vi "initialize timing source.vi"(8 "error in":errorcluster, 11 "timing source in":refnum<class "usec timing source.lvclass">) -> (0 "error out":errorcluster, 3 "timing source out":refnum<class "usec timing source.lvclass">)   [LabVIEW 2013, in "usec timing source.lvclass"]
doc: "An interface for initializing a timing source. In many cases this may be a no-op. There is no expectation about when this function should be called, but it must be called before entering the loop to be timed."
uses:
  usec timing source.lvclass
  usec timing source.lvclass/usec timing source.ctl
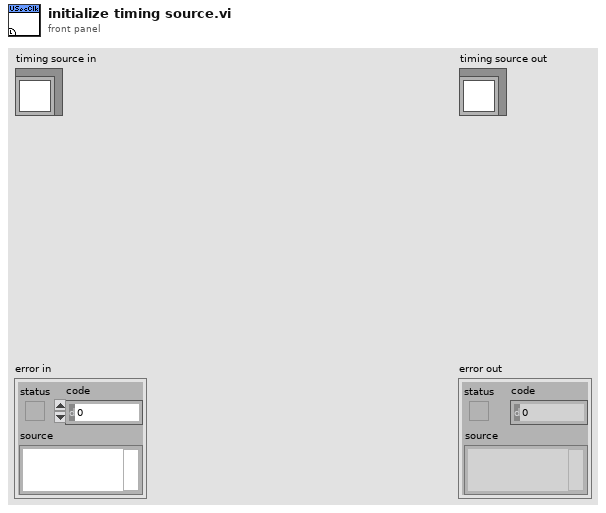
[diagram p1: front panel]
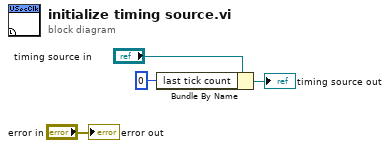
[diagram p0: block diagram]
diagram:
  n1 = Bundle By Name(cluster="timing source in", "last tick count"=u32 0) -> (→"timing source out":refnum<class "usec timing source.lvclass">)
  "error out" <- "error in"
